vi "Numeric Control - Integer.vi"() -> ()   [LabVIEW 2012]
doc: "Sample numeric display item."
uses:
  <vilib>/NI Veristand/Display Template Support/Display Template Support.llb/cluster_Screen Item Settings.ctl
  <vilib>/NI Veristand/Display Template Support/Display Template Support.llb/cluster_Graph Scale Settings.ctl
  <vilib>/NI Veristand/Display Template Support/Display Template Support.llb/cluster_Graph Plot Settings.ctl
  NationalInstruments.VeriStand.SystemStorage
  <vilib>/NI Veristand/Display Template Support/Display Template Support.llb/enum_Display Template Handler Minimal To Widget Msg.ctl
  <vilib>/NI Veristand/Display Template Support/Display Template Support.llb/enum_Display Template Handler Minimal To Workspace.ctl
  Integer Object Parameters.ctl
  <vilib>/NI Veristand/Execution/Workspace/NI_VS Workspace ExecutionAPI.lvlib
panel:
  in  "NIVS.System Definition Root":refnum<k24>
  in  "NIVS.Gateway IP Address":string
  in  "Numeric":i64
  out "Label":string="Numeric"
  in  "Item.Data":T1
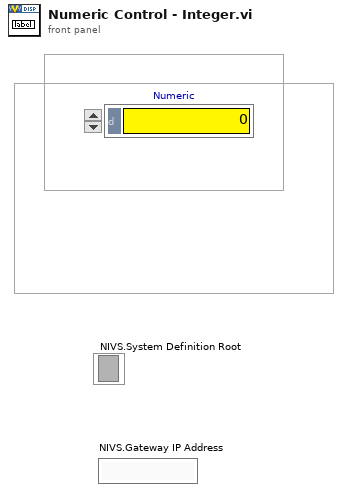
[diagram p1: front panel]
types:
  T1 = typedef "cluster_Screen Item Settings.ctl" = cluster{"Template VI":string, "Position X":i32, "Position Y":i32, "Custom":string, "Show Title Bar":bool, "ID":i32, "Always On Top":bool, "Allow Resize":bool, "Allow Minimize":bool, "Allow Close":bool, "Size to Screen":bool, "Screen.ID":i32, "State":enum16{"Normal", "New"}, "Title":string, "Window Bounds":cluster{"[0]":i16, "[1]":i16, "[2]":i16, "[3]":i16}, "Channel Ref":u64, "Unit":string, "Default Units?":bool, "Flash Limit?":bool, "Color 1":u32, "Color 2":u32, "Color 3":u32, "Color 4":u32, "Bck Color":u32, "Fore Color":u32, "Limit 1":dbl, "Limit 2":dbl, "Limit 3":dbl, "Limit 4":dbl, "Limit Mode 1":i32, "Limit Mode 2":i32, "Limit Mode 3":i32, "Limit Mode 4":i32, "Scale Precision":i32, "Scale Min":dbl, "Scale Max":dbl, "Format":i32, "Precision":i32, "Background Type":i32, "IDs":i32[], "Units":string[], "Labels":string[], "Scale Factor":dbl, "Scale Offset":dbl, "YScale Index":u32[], "XScale":T2, "YScales":T2[], "Plots":T3[], "Update Period":dbl, "History Length":dbl, "My.Ref":refnum<vi>, "Is Control?":bool, "Channel Paths":string[], "Custom Data":variant}
  T2 = typedef "cluster_Graph Scale Settings.ctl" = cluster{"Format":u8, "Precision":u8, "Fit":u8, "Label":string, "Use Default Label":bool, "Label Visible":bool, "Min":dbl, "Max":dbl}
  T3 = typedef "cluster_Graph Plot Settings.ctl" = cluster{"Bar Style":u8, "Fill To":i16, "Fill/PtColor":u32, "Line Style":u8, "Line Width":u8, "Color":u32, "Interp":u8, "Point Style":u8}
  T4 = typedef "enum_Display Template Handler Minimal To Workspace.ctl" = cluster{"Operation":enum16{"SetCustomData", "DeleteItem"}, "Data":variant}
  T5 = typedef "enum_Display Template Handler Minimal To Widget Msg.ctl" = enum16{"Stop", "LaunchConfigDialog"}
  T6 = typedef "Integer Object Parameters.ctl" = cluster{"Node Path":string, "NodePathArray":string[], "Integer":cluster{"Label":string, "Digits of Precision":u8, "Integer Format":enum8{"Decimal", "Scientific", "Engineering", "Binary", "Octal", "Hexadecimal", "Relative Time", "Time and Date", "SI"}}}
  T7 = enum8{"Decimal", "Scientific", "Engineering", "Binary", "Octal", "Hexadecimal", "Relative Time", "Time and Date", "SI"}
  T8 = typedef "NI_VS Workspace ExecutionAPI.lvlib/WorkspaceAPI.ctl" = refnum<k24>
  T9 = cluster{"Node Path":string, "NodePathArray":string[], "Integer":cluster{"Label":string, "Digits of Precision":u8, "Integer Format":enum8{"Decimal", "Scientific", "Engineering", "Binary", "Octal", "Hexadecimal", "Relative Time", "Time and Date", "SI"}}}
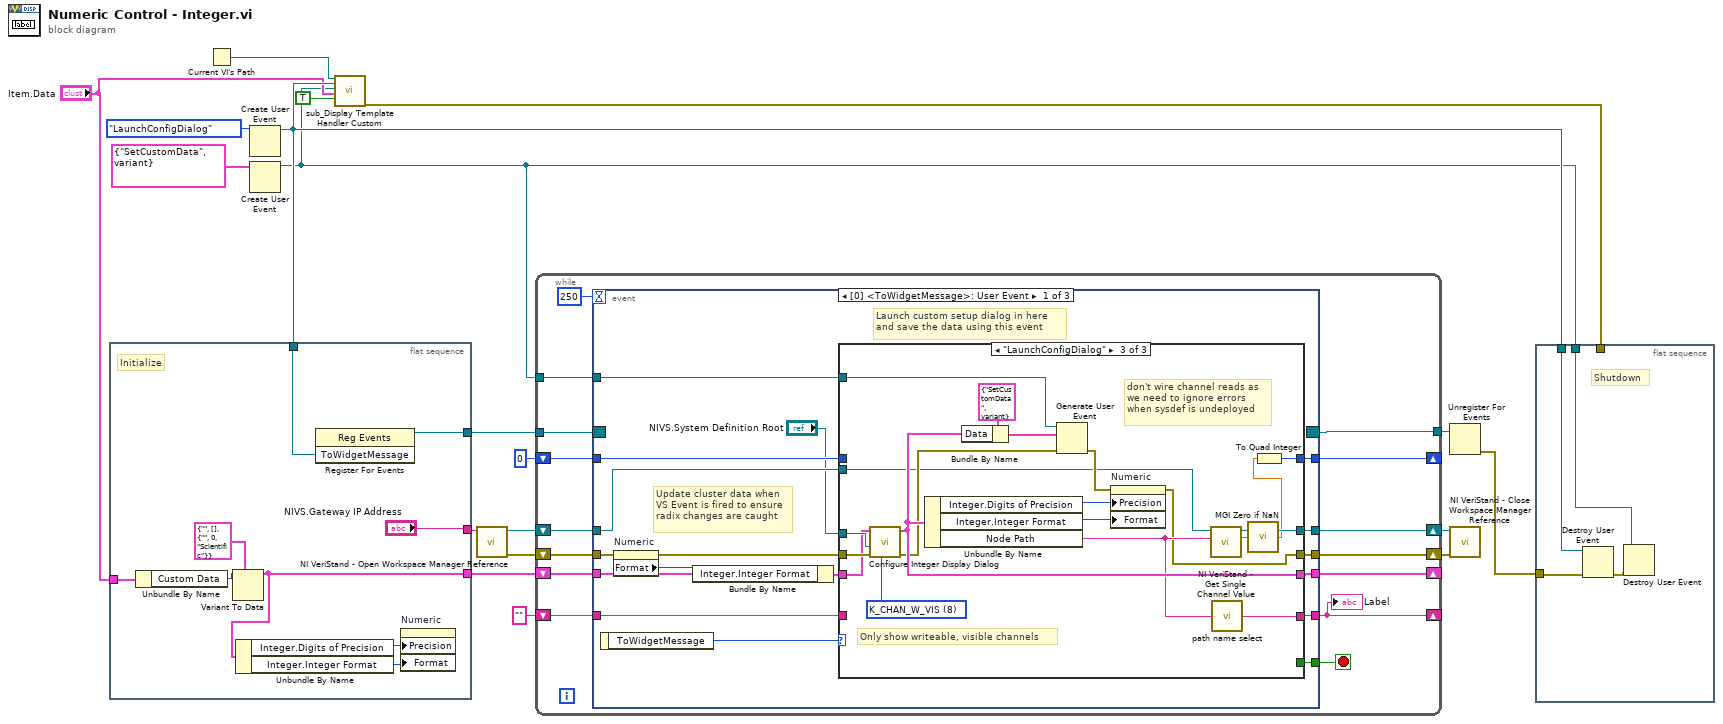
[diagram p0: block diagram]
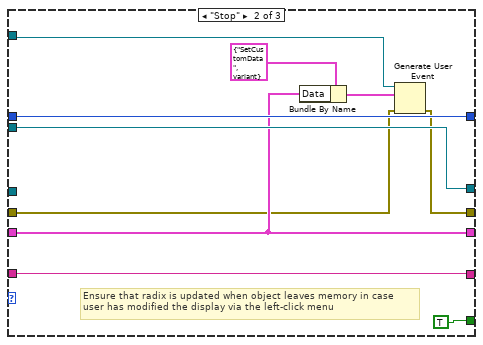
[diagram p3: hidden frame]
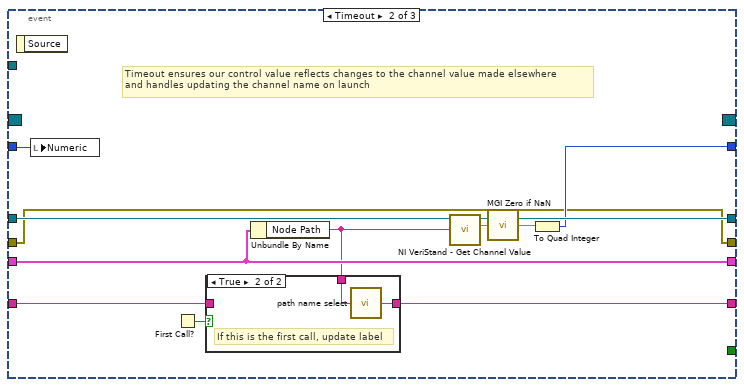
[diagram p4: hidden frame]
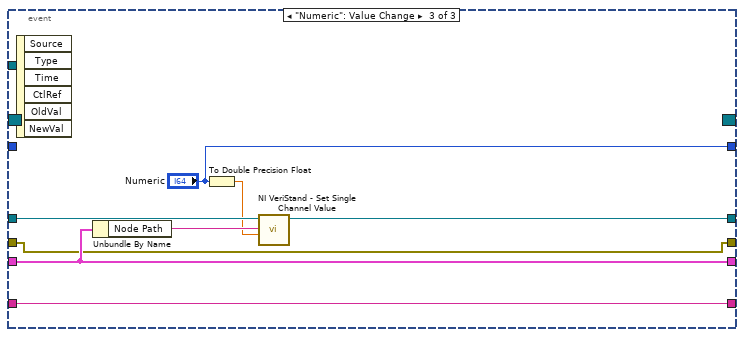
[diagram p6: hidden frame]
diagram:
  n1 = flat-sequence {
    tunnel: [w28] -> w17
    tunnel: w14 -> [w27]
    tunnel: "Item.Data" -> [w26]
    tunnel: [w22] -> w8
    tunnel: ["NIVS.Gateway IP Address"] -> w3
    frame #0 {
      # "Initialize"
      n2 = Unbundle By Name(w26) -> ("Custom Data"=w25:variant)
      n3 = Variant To Data(type=T6 {"Node Path"="", "NodePathArray"=[], "Integer"={"Label"="", "Digits of Precision"=0, "Integer Format"=enum."Scientific"}}, Variant=w25) -> (data=w22:T6)  [unwired: 1 in, 1 out]
      n4 = Unbundle By Name(w22) -> ("Integer.Digits of Precision"=w21:u8, "Integer.Integer Format"=w20:T7)
      n5 = register-events(w27) -> (reference out=w28:refnum<event-registration>)  [unwired: 2 in, 1 out]
      n6 = property on="Numeric" class="DigNum (strict)"("Precision"=w21, "Format"=w20) -> ()  [unwired: 2 in, 2 out]
    }
  }
  n7 = Current VI's Path() -> (path=w12:path)
  n8 = Create User Event(user event datatype=enum_Display_Template_Handler_Minimal_To_Widget_Msg."LaunchConfigDialog" ("ToWidgetMessage")) -> (user event=w14:refnum<user-event>)  [unwired: 1 in, 1 out]
  n9 = Create User Event(user event datatype=T4 {"Operation"=enum."SetCustomData", "Data"=variant} ("Data")) -> (user event=w10:refnum<user-event>)  [unwired: 1 in, 1 out]
  n10 = call <vilib>:"sub_Display Template Handler Custom.vi"("Parent.Path"=w12, "ToWidgetEvent"=w14, "ToWorkspace"=w10, "Item.Data"="Item.Data", "Resizable"=TRUE) -> ("error out"=w19:errorcluster)  [unwired: 14 in]
  n11 = call <vilib>:"NI VeriStand - Open Workspace Manager Reference.vi"("Gateway IP Address (\"\": localhost)"=w3) -> ("error out"=w6:errorcluster, "WorkspaceManager"=w7:T8)  [unwired: 9 in]
  n12 = while {
    tunnel: w17 -> [w43]
    tunnel: [w41] -> w16
    tunnel: w10 -> [w40]
    shift-right: [w33] -> _
    shift-left: w8 -> [w39]
    shift-right: [w35] -> w5
    shift-left: w7 -> [w37]
    shift-right: [w29] -> w4
    shift-left: w6 -> [w36]
    shift-right: [w30] -> _
    shift-left: i64 0 ("Numeric") -> [w34]
    shift-right: [w31] -> _
    shift-left: "" ("Out") -> [w32]
    stop <- w42 stop-if-true
    n13 = event shown="[0] <ToWidgetMessage>: User Event" {
      selector: w43 -> [_ _ _]
      dyn-events: [_ _ _] -> w41
      timeout: 250 -> [_ _ _]
      tunnel: [w59 _ _] -> w42
      tunnel: w40 -> [w58 _ _]
      tunnel: [w57 w103 w115] -> w33
      tunnel: w39 -> [w45 w103 w115]
      tunnel: [w56 w101 "Numeric"] -> w30
      tunnel: w37 -> [w55 w104 w118]
      tunnel: w36 -> [w47 w98 w111]
      tunnel: [w54 w102 w116] -> w35
      tunnel: [w53 w98 w111] -> w29
      tunnel: w34 -> [w52 w100 _]
      tunnel: [w51 w105 w114] -> w31
      tunnel: w32 -> [w50 w106 w114]
      event User Event {
        # "Update cluster data when\nVS Event is fired to ensure\nradix changes are caught"
        # "Launch custom setup dialog in here\nand save the data using this event"
        n14 = event-data() -> ("ToWidgetMessage"=w60:T5)  [unwired: 1 out]
        n15 = property on="Numeric" class="DigNum (strict)"(error in=w47) -> (error out=w48:errorcluster, "Format"=w49:u8)  [unwired: 1 in, 1 out]
        n16 = Bundle By Name(cluster=w45, "Integer.Integer Format"=w49) -> (w46:T6)
        n17 = case shown="\"LaunchConfigDialog\"" w60 {
          tunnel: [_ TRUE _] -> w59
          tunnel: w58 -> [_ w69 w95]
          tunnel: [w65 w67 w89] -> w57
          tunnel: w46 -> [w65 w67 w90]
          tunnel: [w62 w73 w80] -> w56
          tunnel: w55 -> [w64 w74 w83]
          tunnel: w48 -> [w63 w66 w92]
          tunnel: [w64 w74 w81] -> w54
          tunnel: [w63 w68 w78] -> w53
          tunnel: w52 -> [w62 w73 _]
          tunnel: "NIVS.System Definition Root" -> [_ _ w91]
          tunnel: [w61 w72 w84] -> w51
          tunnel: w50 -> [w61 w72 _]
          frame Default {
          }
          frame "Stop" {
            # "Ensure that radix is updated when object leaves memory in case\nuser has modified the display via the left-click menu"
            n18 = Bundle By Name(cluster=T4 {"Operation"=enum."SetCustomData", "Data"=variant} ("event data"), "Data"=w67) -> (w70:T4)
            n19 = Generate User Event(user event=w69, event data cluster=w70, error in=w66) -> (error out=w68:errorcluster)  [unwired: 1 out]
          }
          frame "LaunchConfigDialog" {
            w79 = u8 8 items=["K_CHAN_R", "K_CHAN_W", "K_CHAN_RW", "K_CHAN_VOLT", "K_CHAN_FAULT", "K_ALL", "K_CUSTOM", "K_CHAN_R_VIS", "K_CHAN_W_VIS", "K_CHAN_RW_VIS", "K_CHAN_VOLT_VIS", "K_CHAN_FAULT_VIS"] ("DisplayFilter")
            # "Only show writeable, visible channels"
            # "don't wire channel reads as\nwe need to ignore errors\nwhen sysdef is undeployed"
            n20 = call "Configure Integer Display Dialog.vi"("DisplayFilter"=w79, "error in (no error)"=w92, "NIVS.System Definition Root"=w91, "Data cluster in"=w90) -> ("error out"=w86:errorcluster, "Data cluster out"=w89:T9)  [unwired: 6 in]
            n21 = Unbundle By Name(w89) -> ("Integer.Digits of Precision"=w88:u8, "Integer.Integer Format"=w87:T7, "Node Path"=w82:string)
            n22 = Bundle By Name(cluster=T4 {"Operation"=enum."SetCustomData", "Data"=variant} ("event data"), "Data"=w89) -> (w93:T4)
            n23 = Generate User Event(user event=w95, event data cluster=w93, error in=w86) -> (error out=w85:errorcluster)  [unwired: 1 out]
            n24 = property on="Numeric" class="DigNum (strict)"(error in=w85, "Precision"=w88, "Format"=w87) -> (error out=w78:errorcluster)  [unwired: 1 in, 1 out]
            n25 = call <vilib>:"NI VeriStand - Get Single Channel Value.vi"("Channel"=w82, "WorkspaceManager in"=w83) -> ("Value"=w77:dbl, "WorkspaceManager out"=w81:T8)  [unwired: 7 in, 1 out]
            n26 = call "path name select.vi"("In"=w82) -> ("Out"=w84:string)
            n27 = call <userlib>:"MGI Zero if NaN.vi"("Number In"=w77) -> ("Number Out"=w76:dbl)
            n28 = To Quad Integer(1:w76) -> (0:w80:i64)
          }
        }
      }
      event Timeout {
        # "Timeout ensures our control value reflects changes to the channel value made elsewhere\nand handles updating the channel name on launch"
        n29 = event-data() -> ()  [unwired: 2 out]
        n30 = local write "Numeric"(w100) -> ()
        n31 = First Call?() -> (First Call?: T/F=w107:bool)
        n32 = Unbundle By Name(w103) -> ("Node Path"=w99:string)
        n33 = case shown="True" w107 {
          tunnel: w106 -> [w108 _]
          tunnel: [w108 w110] -> w105
          tunnel: w99 -> [_ w109]
          frame False {
          }
          frame True {
            # "If this is the first call, update label"
            n34 = call "path name select.vi"("In"=w109) -> ("Out"=w110:string)
          }
        }
        n35 = call-poly <vilib>:"NI VeriStand - Get Channel Value.vi"("Channel"=w99, "WorkspaceManager in"=w104) -> ("Value"=w97:dbl, "WorkspaceManager out"=w102:T8)  [unwired: 7 in, 1 out]
        n36 = call <userlib>:"MGI Zero if NaN.vi"("Number In"=w97) -> ("Number Out"=w96:dbl)
        n37 = To Quad Integer(1:w96) -> (0:w101:i64)
      }
      event "Numeric": Value Change {
        n38 = event-data() -> ()  [unwired: 7 out]
        n39 = Unbundle By Name(w115) -> ("Node Path"=w117:string)
        n40 = To Double Precision Float(number="Numeric") -> (double precision float=w113:dbl)
        n41 = call <vilib>:"NI VeriStand - Set Single Channel Value.vi"("Value"=w113, "Channel"=w117, "WorkspaceManager in"=w118) -> ("WorkspaceManager out"=w116:T8)  [unwired: 7 in, 1 out]
      }
    }
    "Label" <- w31
  }
  n42 = Unregister For Events(event registration refnum=w16) -> (error out=w15:errorcluster)  [unwired: 1 in]
  n43 = call <vilib>:"NI VeriStand - Close Workspace Manager Reference.vi"("error in (no error)"=w4, "WorkspaceManager"=w5) -> ()  [unwired: 9 in, 1 out]
  n44 = flat-sequence {
    tunnel: w19 -> [_]
    tunnel: w15 -> [w121]
    tunnel: w14 -> [w122]
    tunnel: w10 -> [w119]
    frame #0 {
      # "Shutdown"
      n45 = Destroy User Event(user event=w122, error in=w121) -> (error out=w120:errorcluster)
      n46 = Destroy User Event(user event=w119, error in=w120) -> ()  [unwired: 1 out]
    }
  }
